vi "EnterOrExitBySearch1DArray.vi"(8 "In (T) / Out (F)":bool=TRUE, 9 "Occup array":refnum<vi>[](array[refnum]), 10 "Sense array":refnum<vi>[](array[refnum]), 11 "Occupancy in":T2) -> (3 "Occupancy out":T1)   [LabVIEW 2024]
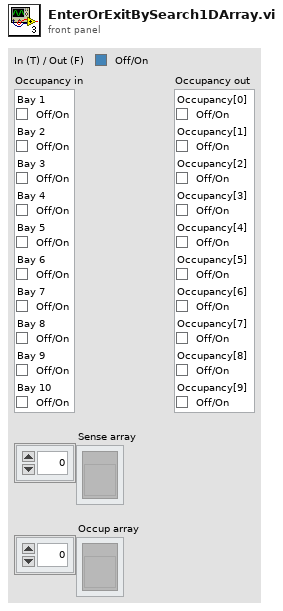
[diagram p1: front panel]
types:
  T1 = cluster{"Occupancy[0]":bool, "Occupancy[1]":bool, "Occupancy[2]":bool, "Occupancy[3]":bool, "Occupancy[4]":bool, "Occupancy[5]":bool, "Occupancy[6]":bool, "Occupancy[7]":bool, "Occupancy[8]":bool, "Occupancy[9]":bool}
  T2 = cluster{"Bay 1":bool, "Bay 2":bool, "Bay 3":bool, "Bay 4":bool, "Bay 5":bool, "Bay 6":bool, "Bay 7":bool, "Bay 8":bool, "Bay 9":bool, "Bay 10":bool}
  T3 = cluster{"Occupancy in[0]":bool, "Occupancy in[1]":bool, "Occupancy in[2]":bool, "Occupancy in[3]":bool, "Occupancy in[4]":bool, "Occupancy in[5]":bool, "Occupancy in[6]":bool, "Occupancy in[7]":bool, "Occupancy in[8]":bool, "Occupancy in[9]":bool}
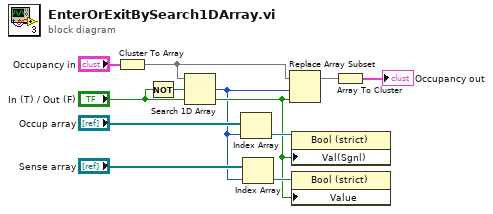
[diagram p0: block diagram]
diagram:
  n1 = Cluster To Array(cluster="Occupancy in") -> (array=w4:bool[])
  n2 = Not(x="In (T) / Out (F)") -> (.not. x?=w2:bool)
  n3 = Search 1D Array(1D array=w4, element=w2) -> (index of element=w1:i32)  [unwired: 1 in]
  n4 = Index Array(array="Occup array", index=w1) -> (element=w7:refnum<vi>)
  n5 = Index Array(array="Sense array", index=w1) -> (element=w5:refnum<vi>)
  n6 = Replace Array Subset(array=w4, new element="In (T) / Out (F)", index=w1) -> (w9:bool[])
  n7 = property class="Bool (strict)"(reference=w7, "Val(Sgnl)"="In (T) / Out (F)") -> ()  [unwired: 1 in, 2 out]
  n8 = property class="Bool (strict)"(reference=w5, "Value"="In (T) / Out (F)") -> ()  [unwired: 1 in, 2 out]
  n9 = Array To Cluster(array=w9) -> (cluster=→"Occupancy out":T3)
